vi "Set Protocol.vi"(8 "error in (no error)":errorcluster, 10 "protocol":refnum<class "Protocol Parent.lvclass">, 11 "instrument addon refnum in":T1 format="%.0x") -> (0 "error out":errorcluster, 3 "instrument addon refnum out":T1=18446744073709551615 format="%.0x")   [LabVIEW 2020, in "Instrument Addon Scripting API.lvlib"]
doc: "Sets the protocol object for the specified Instrument Addon Custom Device.\n \nThe input protocol must be a child of the protocol's parent class. It is formatted as one of the following classes: TCP.lvclass, UDP.lvclass, VISA.lvclass, RS-xxx.lvclass, AK TCP.lvclass, AK RS-xxx.lvclass, RS-xxx to GPIB ConvBox.lvclass"
uses:
  Instrument Addon Scripting API.lvlib
  <vilib>/NI VeriStand/Custom Device API/Custom Device Item Ref.ctl
  Libraries Directory/Protocols.lvlibp/Protocol Parent/Protocol Parent.lvclass
  Libraries Directory/Protocols.lvlibp/RS-xxx/RS-xxx.lvclass
  Shared Directory/RSXXX Port Settings.ctl
  Shared Directory/FG Control.ctl
  Libraries Directory/Protocols.lvlibp/AK RS-xxx/AK RS-xxx.lvclass
  Libraries Directory/Protocols.lvlibp/UDP/UDP.lvclass
  Shared Directory/UDP Settings.ctl
  Libraries Directory/Protocols.lvlibp/TCP/TCP.lvclass
  Shared Directory/TCPIP Settings.ctl
  Libraries Directory/Protocols.lvlibp/AK TCP/AK TCP.lvclass
  Libraries Directory/Protocols.lvlibp/VISA/VISA.lvclass
  Shared Directory/VISA Settings.ctl
  Libraries Directory/Protocols.lvlibp/RS-xxx to GPIB ConvBox/RS-xxx to GPIB ConvBox.lvclass
  Shared Directory/GPIB ConvBox Settings.ctl
  Libraries Directory/Protocols.lvlibp/RS-xxx/Data Access/Read PortSettings.vi
  Shared Directory/Constants.vi
  <vilib>/NI VeriStand/Custom Device API/NI VeriStand - Get Item Property.vi
  <vilib>/NI VeriStand/Custom Device API/Get Item Property (String).vi
  <vilib>/NI VeriStand/Custom Device API/Get Item Property (U32).vi
  <vilib>/NI VeriStand/Custom Device API/Get Item Property (Boolean).vi
  <vilib>/NI VeriStand/Custom Device API/NI VeriStand - Set Item Property.vi
  <vilib>/NI VeriStand/Custom Device API/Set Item Property (String).vi
  <vilib>/NI VeriStand/Custom Device API/Set Item Property (U32).vi
  <vilib>/NI VeriStand/Custom Device API/Set Item Property (Boolean).vi
  Dependencies.llb/Instrument_Addon_Scripting_Dependencies_SysDef.Property.Get.vi
  Dependencies.llb/Instrument_Addon_Scripting_Dependencies_SysDef.Property.Get.String.vi
  Dependencies.llb/Instrument_Addon_Scripting_Dependencies_SysDef.Property.Set.vi
  Dependencies.llb/Instrument_Addon_Scripting_Dependencies_SysDef.Property.Set.String.vi
  Libraries Directory/Protocols.lvlibp/UDP/Data Access/Read Local IP Address.vi
  Libraries Directory/Protocols.lvlibp/UDP/Data Access/Read Local Port.vi
  Libraries Directory/Protocols.lvlibp/UDP/Data Access/Read Target IP Address.vi
  Libraries Directory/Protocols.lvlibp/UDP/Data Access/Read Target Port.vi
  Libraries Directory/Protocols.lvlibp/TCP/Data Access/Read IP Address.vi
  Libraries Directory/Protocols.lvlibp/TCP/Data Access/Read Port.vi
  Libraries Directory/Protocols.lvlibp/VISA/Data Access/Read Append Write Termination Character.vi
  Libraries Directory/Protocols.lvlibp/VISA/Data Access/Read Enable Termination Character.vi
  Libraries Directory/Protocols.lvlibp/VISA/Data Access/Read Termination Character.vi
  Libraries Directory/Protocols.lvlibp/VISA/Data Access/Read Timeout.vi
  Libraries Directory/Protocols.lvlibp/VISA/Data Access/Read VISA Resource.vi
  Libraries Directory/Protocols.lvlibp/RS-xxx to GPIB ConvBox/Data Access/Read Assert Ren with IFC.vi
  Libraries Directory/Protocols.lvlibp/RS-xxx to GPIB ConvBox/Data Access/Read ConvBox Address.vi
  Libraries Directory/Protocols.lvlibp/RS-xxx to GPIB ConvBox/Data Access/Read GPIB Address.vi
  Libraries Directory/Protocols.lvlibp/RS-xxx to GPIB ConvBox/Data Access/Read IST bit sense.vi
  Libraries Directory/Protocols.lvlibp/RS-xxx to GPIB ConvBox/Data Access/Read Port.vi
  Libraries Directory/Protocols.lvlibp/RS-xxx to GPIB ConvBox/Data Access/Read System controller.vi
  Shared Directory/Instrument Addon Shared.lvlib
  <vilib>/NI VeriStand/Custom Device API/Custom Device API.lvlib
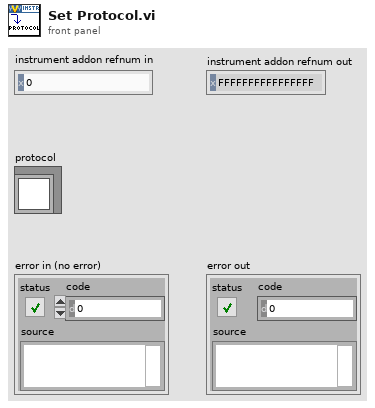
[diagram p1: front panel]
types:
  T1 = typedef "Custom Device API.lvlib/Custom Device Item Ref.ctl" = u64
  T2 = typedef "Instrument Addon Shared.lvlib/FG Control.ctl" = enum16{"Get", "Set"}
  T3 = typedef "Instrument Addon Shared.lvlib/RSXXX Port Settings.ctl" = cluster{"Port":string, "Baud Rate":u32, "Data Bits":u16, "Parity":enum16{"None", "Odd", "Even", "Mark", "Space"}, "Stop Bits":u16, "Flow Control":u16, "XON":enum16{"NUL", "SOH", "STX", "ETX", "EOT", "ENQ", "ACK", "BEL", "BS", "HT", "LF", "VT", "FF", "CR", "SO", "SI", "DLE", "DC1", "DC2", "DC3", "DC4", "NAK", "SYN", "ETB", "CAN", "EM", "SUB", "ESC", "FS", "GS", "RS", "US", "SP", "!", "\"", "#", "$", "%", "&", "'", "(", ")", "*", "+", ",", "- (-)", ".", "/", "0", "1", "2", "3", "4", "5", "6", "7", "8", "9", ":", ";", "<", "=", ">", "?", "@", "A", "B", "C", "D", "E", "F", "G", "H", "I", "J", "K", "L", "M", "N", "O", "P", "Q", "R", "S", "T", "U", "V", "W", "X", "Y", "Z", "[", "\\", "]", "^", "_", "`", "a", "b", "c", "d", "e", "f", "g", "h", "i", "j", "k", "l", "m", "n", "o", "p", "q", "r", "s", "t", "u", "v", "w", "x", "y", "z", "{", "|", "}", "~"}, "XOFF":enum16{"NUL", "SOH", "STX", "ETX", "EOT", "ENQ", "ACK", "BEL", "BS", "HT", "LF", "VT", "FF", "CR", "SO", "SI", "DLE", "DC1", "DC2", "DC3", "DC4", "NAK", "SYN", "ETB", "CAN", "EM", "SUB", "ESC", "FS", "GS", "RS", "US", "SP", "!", "\"", "#", "$", "%", "&", "'", "(", ")", "*", "+", ",", "- (-)", ".", "/", "0", "1", "2", "3", "4", "5", "6", "7", "8", "9", ":", ";", "<", "=", ">", "?", "@", "A", "B", "C", "D", "E", "F", "G", "H", "I", "J", "K", "L", "M", "N", "O", "P", "Q", "R", "S", "T", "U", "V", "W", "X", "Y", "Z", "[", "\\", "]", "^", "_", "`", "a", "b", "c", "d", "e", "f", "g", "h", "i", "j", "k", "l", "m", "n", "o", "p", "q", "r", "s", "t", "u", "v", "w", "x", "y", "z", "{", "|", "}", "~"}, "End Read on Termination Character":bool, "End Write on Termination Character":bool, "Termination Character":u8}
  T4 = typedef "Instrument Addon Shared.lvlib/UDP Settings.ctl" = cluster{"Local IP Address":string, "Local Port":u16, "Target IP Address":string, "Target Port":u16}
  T5 = typedef "Instrument Addon Shared.lvlib/TCPIP Settings.ctl" = cluster{"IP Address":string, "Port":u16}
  T6 = typedef "Instrument Addon Shared.lvlib/VISA Settings.ctl" = cluster{"VISA Resource":string, "Enable Termination Character":bool, "Termination Character":u8, "Timeout":u32, "Append Write Termination Character":bool}
  T7 = typedef "Instrument Addon Shared.lvlib/GPIB ConvBox Settings.ctl" = cluster{"Port":string, "ConvBox Address":string, "Assert Ren with IFC":bool, "System controller":bool, "IST bit sense":bool, "GPIB Address":string}
  T8 = typedef "Protocols.lvlibp/Protocol Parent.lvclass/Base Protocol Type.ctl" = enum16{"RS-XXX", "VISA", "TCPIP", "UDP", "GPIB ConvBox"}
  T9 = cluster{"Port":string, "Baud Rate":u32, "Data Bits":u16, "Parity":enum16{"None", "Odd", "Even", "Mark", "Space"}, "Stop Bits":u16, "Flow Control":u16, "XON":enum16{"NUL", "SOH", "STX", "ETX", "EOT", "ENQ", "ACK", "BEL", "BS", "HT", "LF", "VT", "FF", "CR", "SO", "SI", "DLE", "DC1", "DC2", "DC3", "DC4", "NAK", "SYN", "ETB", "CAN", "EM", "SUB", "ESC", "FS", "GS", "RS", "US", "SP", "!", "\"", "#", "$", "%", "&", "'", "(", ")", "*", "+", ",", "- (-)", ".", "/", "0", "1", "2", "3", "4", "5", "6", "7", "8", "9", ":", ";", "<", "=", ">", "?", "@", "A", "B", "C", "D", "E", "F", "G", "H", "I", "J", "K", "L", "M", "N", "O", "P", "Q", "R", "S", "T", "U", "V", "W", "X", "Y", "Z", "[", "\\", "]", "^", "_", "`", "a", "b", "c", "d", "e", "f", "g", "h", "i", "j", "k", "l", "m", "n", "o", "p", "q", "r", "s", "t", "u", "v", "w", "x", "y", "z", "{", "|", "}", "~"}, "XOFF":enum16{"NUL", "SOH", "STX", "ETX", "EOT", "ENQ", "ACK", "BEL", "BS", "HT", "LF", "VT", "FF", "CR", "SO", "SI", "DLE", "DC1", "DC2", "DC3", "DC4", "NAK", "SYN", "ETB", "CAN", "EM", "SUB", "ESC", "FS", "GS", "RS", "US", "SP", "!", "\"", "#", "$", "%", "&", "'", "(", ")", "*", "+", ",", "- (-)", ".", "/", "0", "1", "2", "3", "4", "5", "6", "7", "8", "9", ":", ";", "<", "=", ">", "?", "@", "A", "B", "C", "D", "E", "F", "G", "H", "I", "J", "K", "L", "M", "N", "O", "P", "Q", "R", "S", "T", "U", "V", "W", "X", "Y", "Z", "[", "\\", "]", "^", "_", "`", "a", "b", "c", "d", "e", "f", "g", "h", "i", "j", "k", "l", "m", "n", "o", "p", "q", "r", "s", "t", "u", "v", "w", "x", "y", "z", "{", "|", "}", "~"}, "End Read on Termination Character":bool, "End Write on Termination Character":bool, "Termination Character":u8}
  T10 = enum16{"NUL", "SOH", "STX", "ETX", "EOT", "ENQ", "ACK", "BEL", "BS", "HT", "LF", "VT", "FF", "CR", "SO", "SI", "DLE", "DC1", "DC2", "DC3", "DC4", "NAK", "SYN", "ETB", "CAN", "EM", "SUB", "ESC", "FS", "GS", "RS", "US", "SP", "!", "\"", "#", "$", "%", "&", "'", "(", ")", "*", "+", ",", "- (-)", ".", "/", "0", "1", "2", "3", "4", "5", "6", "7", "8", "9", ":", ";", "<", "=", ">", "?", "@", "A", "B", "C", "D", "E", "F", "G", "H", "I", "J", "K", "L", "M", "N", "O", "P", "Q", "R", "S", "T", "U", "V", "W", "X", "Y", "Z", "[", "\\", "]", "^", "_", "`", "a", "b", "c", "d", "e", "f", "g", "h", "i", "j", "k", "l", "m", "n", "o", "p", "q", "r", "s", "t", "u", "v", "w", "x", "y", "z", "{", "|", "}", "~"}
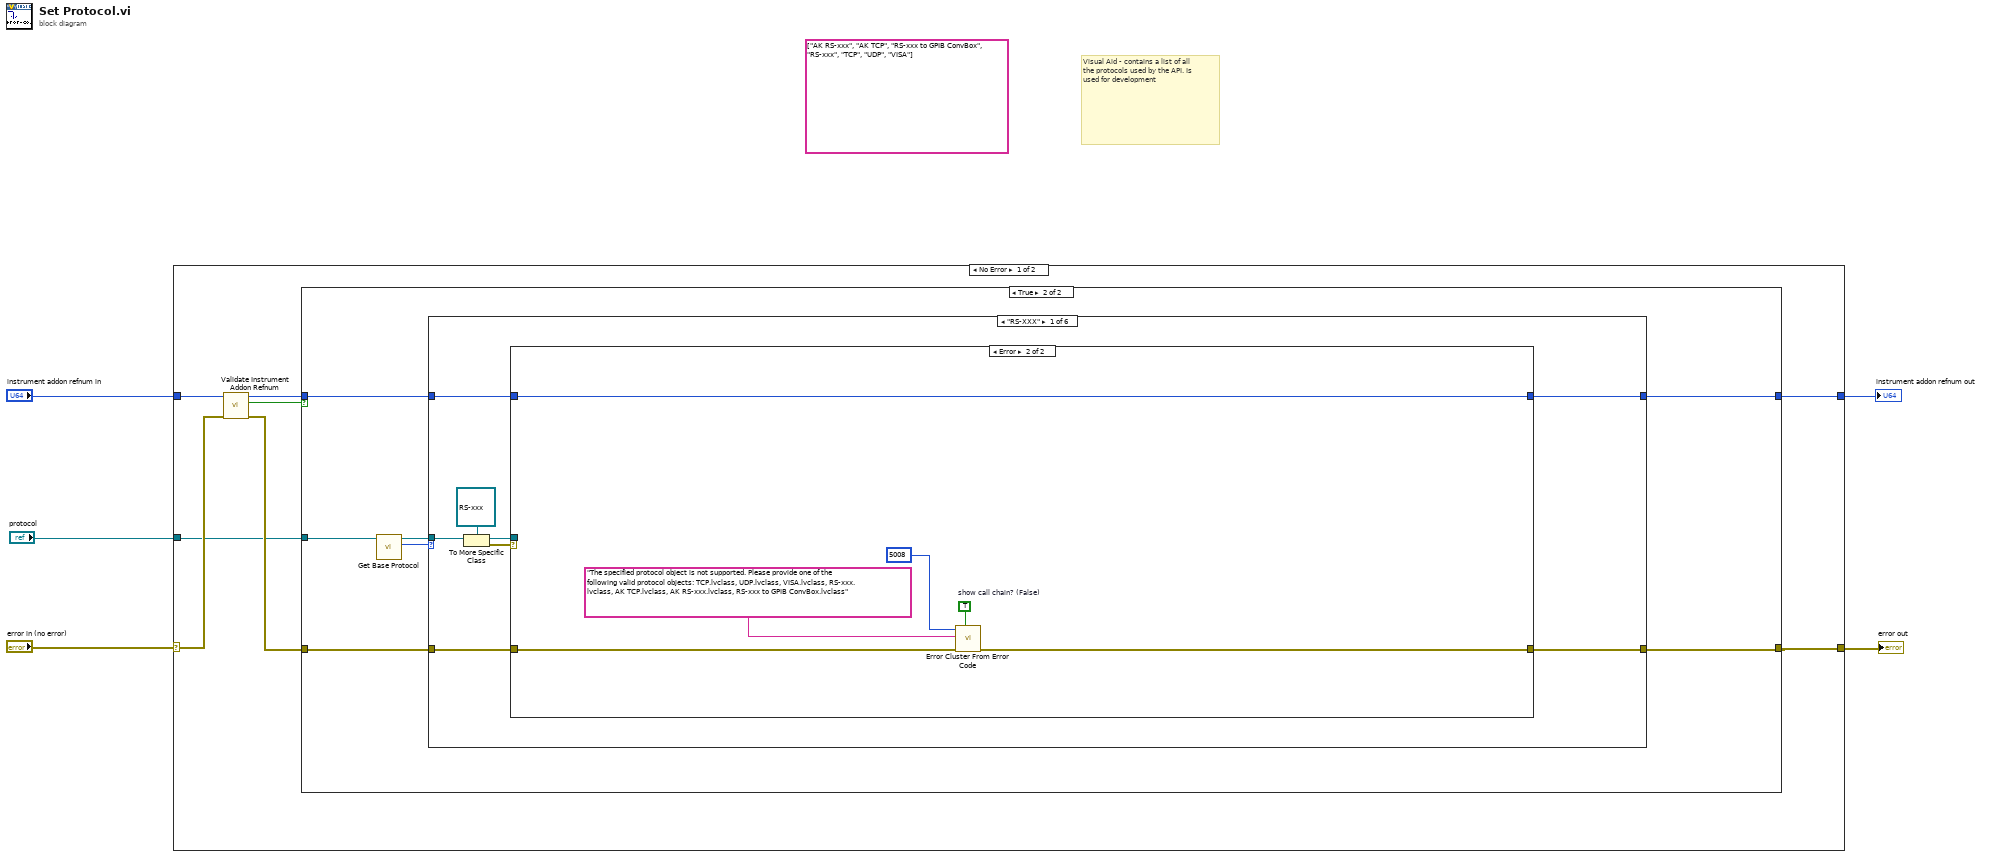
[diagram p0: block diagram]
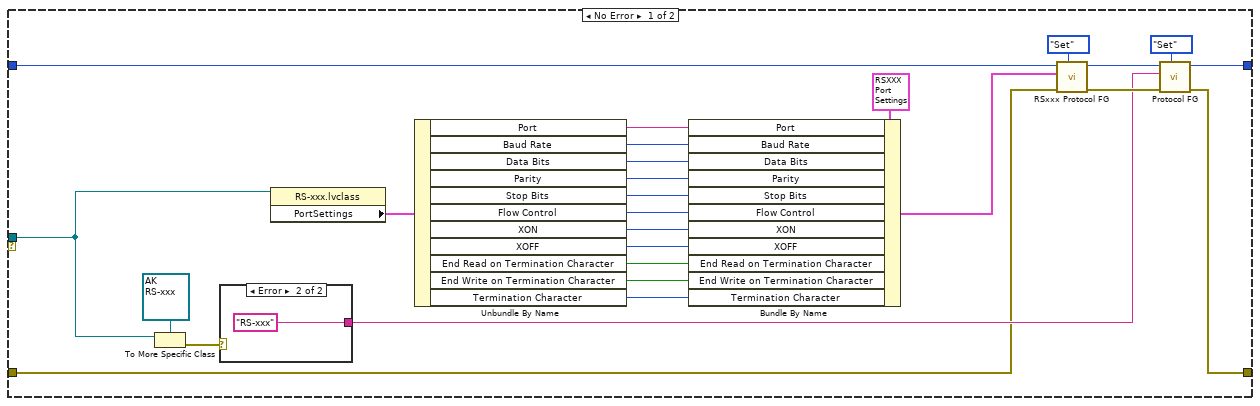
[diagram p3: hidden frame]
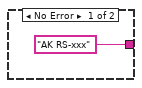
[diagram p4: hidden frame]
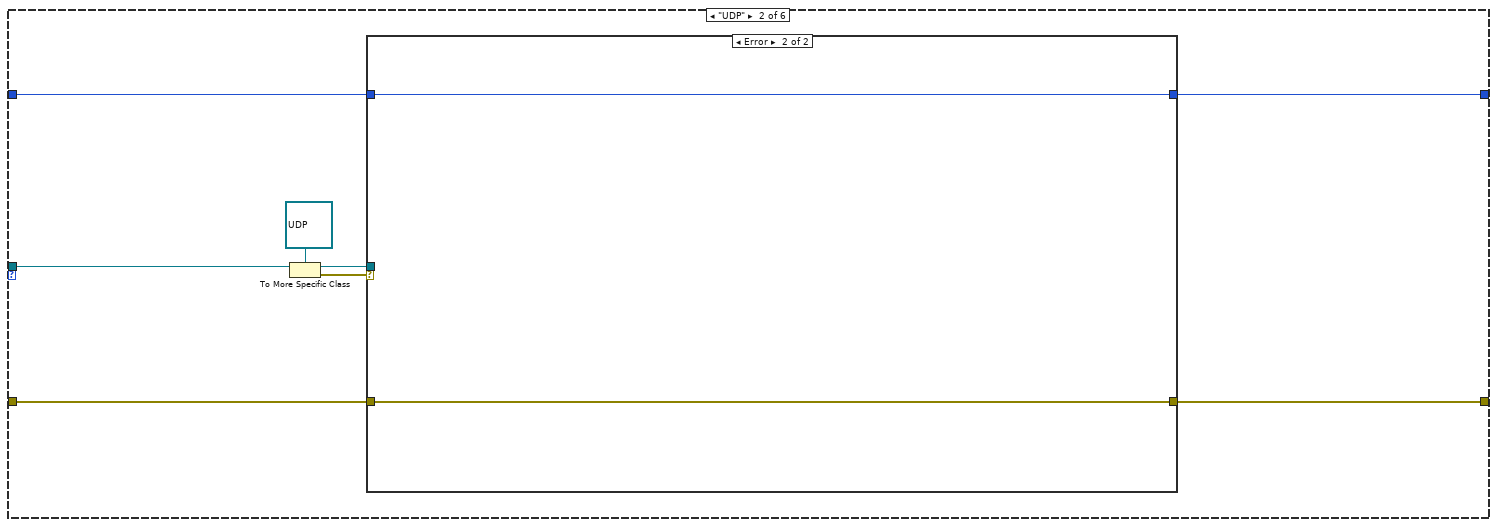
[diagram p5: hidden frame]
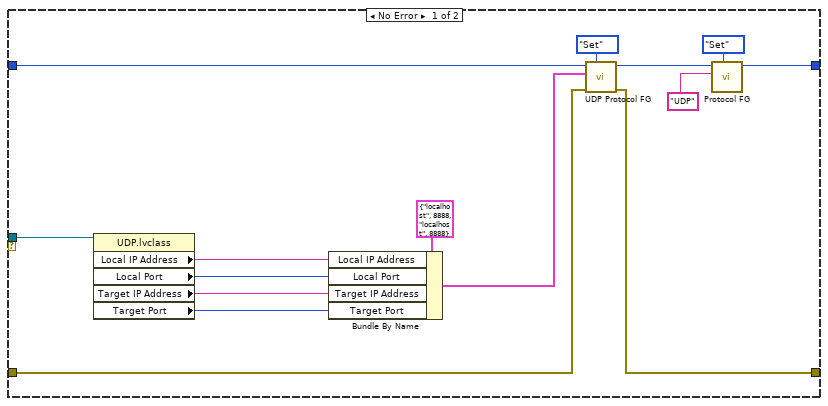
[diagram p6: hidden frame]
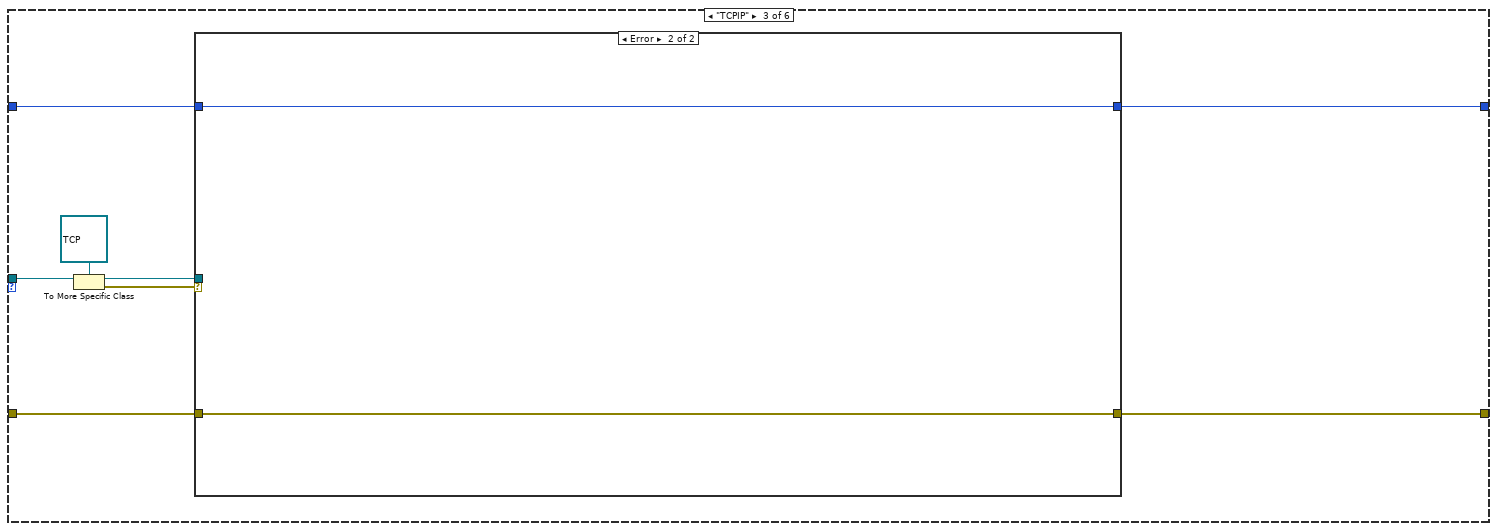
[diagram p7: hidden frame]
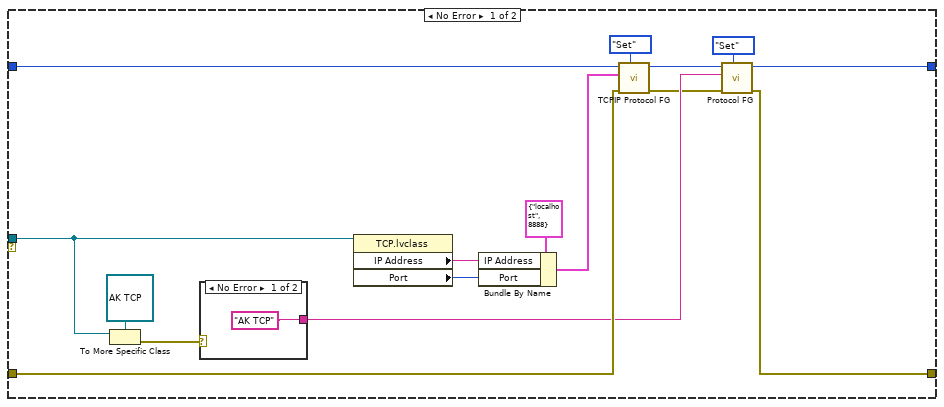
[diagram p8: hidden frame]
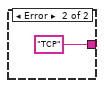
[diagram p9: hidden frame]
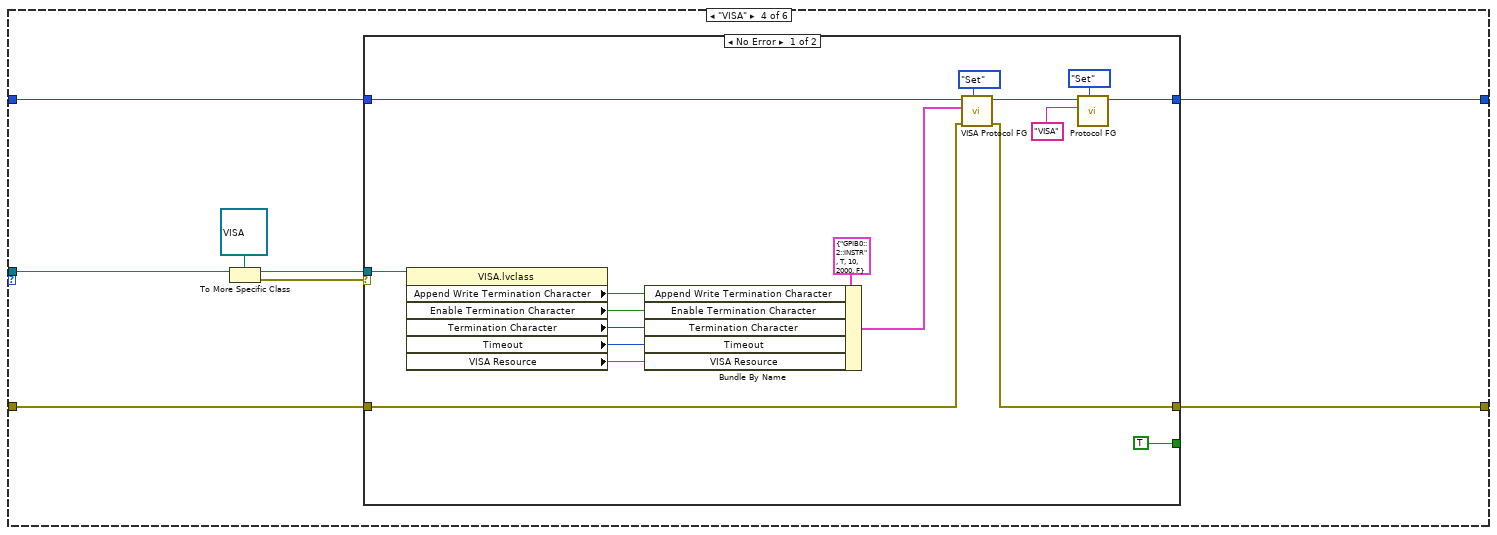
[diagram p10: hidden frame]
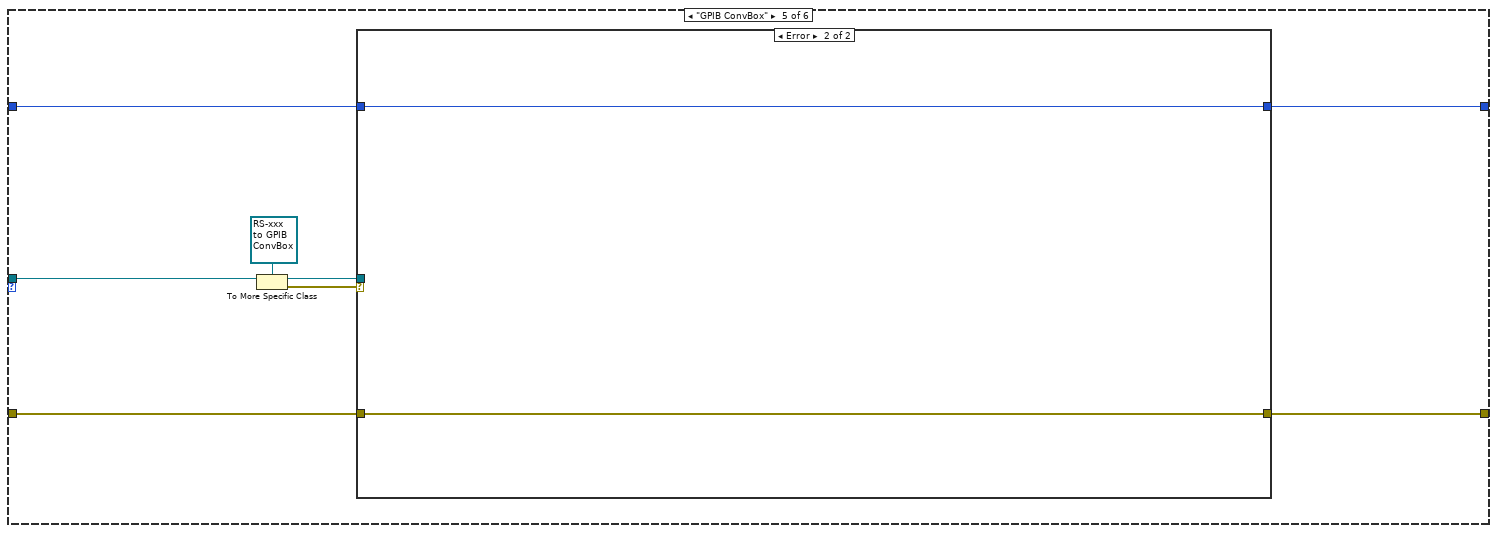
[diagram p12: hidden frame]
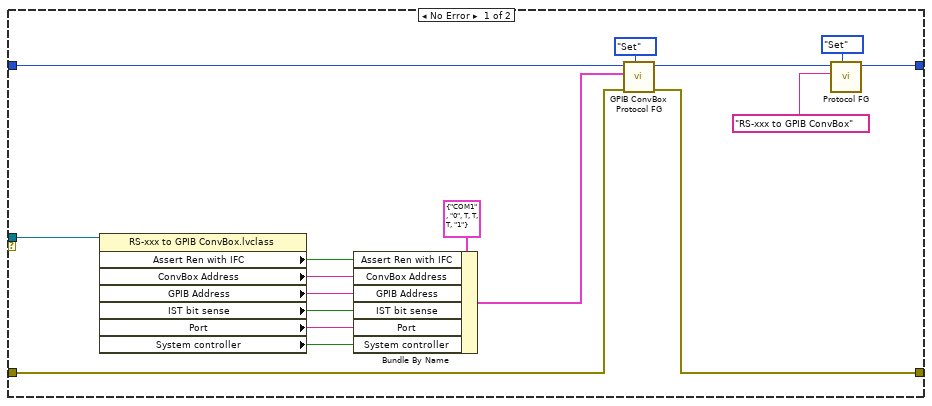
[diagram p13: hidden frame]
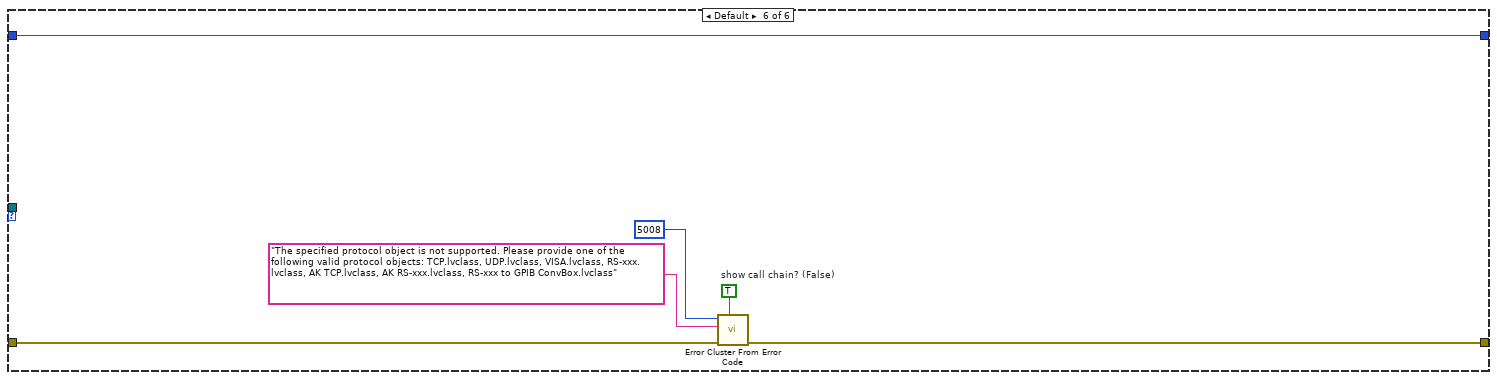
[diagram p14: hidden frame]
diagram:
  (unwired) string[] ["AK RS-xxx", "AK TCP", "RS-xxx to GPIB ConvBox", "RS-xxx", "TCP", "UDP", "VISA"] ("Array")
  # "Visual Aid - contains a list of all the protocols used by the API. Is used for development"
  n1 = case shown="No Error" "error in (no error)" {
    selector: "error in (no error)" -> [w12 w179]
    tunnel: "instrument addon refnum in" -> [w13 w178]
    tunnel: [w9 w179] -> w4
    tunnel: [w8 w178] -> w2
    tunnel: "protocol" -> [w6 _]
    frame No Error {
      n2 = call "Validate Instrument Addon Refnum.vi"("Error In"=w12, "Refnum In"=w13) -> ("Error Out"=w7:errorcluster, "Is Instrument Addon?"=w10:bool, "Refnum Out"=w11:T1)  [unwired: 7 in]
      n3 = case shown="True" w10 {
        tunnel: w11 -> [w15 w21]
        tunnel: [w14 w19] -> w9
        tunnel: [w15 w20] -> w8
        tunnel: w7 -> [w14 w22]
        tunnel: w6 -> [_ w18]
        frame False {
        }
        frame True {
          n4 = call-dynamic "Get Base Protocol.vi"("Protocol Parent in"=w18) -> ("Protocol out"=w16:T8, "Protocol Parent out"=w17:refnum<class "Protocol Parent.lvclass">)  [unwired: 8 in, 1 out]
          n5 = case shown="\"RS-XXX\"" w16 {
            tunnel: w17 -> [w29 w72 w97 w125 w152 _]
            tunnel: w22 -> [w24 w66 w91 w122 w148 w176]
            tunnel: w21 -> [w26 w70 w93 w121 w147 w177]
            tunnel: [w25 w69 w92 w119 w146 w177] -> w20
            tunnel: [w23 w65 w90 w118 w145 w173] -> w19
            frame "RS-XXX" {
              n6 = To More Specific Class(target class=refnum<class "RS-xxx.lvclass"> refnum ("Protocols.lvlibp:RS-xxx.lvclass"), reference=w29) -> (specific class reference=w27:refnum<class "RS-xxx.lvclass">, error out=w28:errorcluster)  [unwired: 1 in]
              n7 = case shown="Error" w28 {
                tunnel: w27 -> [w34 _]
                tunnel: w26 -> [w54 w64]
                tunnel: [w37 w64] -> w25
                tunnel: w24 -> [w31 w61]
                tunnel: [w36 w60] -> w23
                frame No Error {
                  n8 = To More Specific Class(target class=refnum<class "AK RS-xxx.lvclass"> refnum ("Protocols.lvlibp:AK RS-xxx.lvclass"), reference=w34) -> (error out=w33:errorcluster)  [unwired: 1 in, 1 out]
                  n9 = case shown="Error" w33 {
                    tunnel: ["AK RS-xxx" ("filename without extension") "RS-xxx" ("filename without extension")] -> w32
                    frame No Error {
                    }
                    frame Error {
                    }
                  }
                  n10 = property class="RS-xxx.lvclass"(reference=w34) -> ("PortSettings"=w55:T9)  [unwired: 1 in, 2 out]
                  n11 = Unbundle By Name(w55) -> ("Port"=w53:string, "Baud Rate"=w52:u32, "Data Bits"=w51:u16, "Parity"=w50:enum16{"None", "Odd", "Even", "Mark", "Space"}, "Stop Bits"=w49:u16, "Flow Control"=w48:u16, "XON"=w47:T10, "XOFF"=w46:T10, "End Read on Termination Character"=w45:bool, "End Write on Termination Character"=w44:bool, "Termination Character"=w43:u8)
                  n12 = Bundle By Name(cluster=T3 {"Port"="COM1", "Baud Rate"=9600, "Data Bits"=8, "Parity"=enum."None", "Stop Bits"=10, "Flow Control"=0, "XON"=enum."DC1", "XOFF"=enum."DC3", "End Read on Termination Character"=TRUE, "End Write on Termination Character"=TRUE, "Termination Character"=10} ("Serial Config"), "Port"=w53, "Baud Rate"=w52, "Data Bits"=w51, "Parity"=w50, "Stop Bits"=w49, "Flow Control"=w48, "XON"=w47, "XOFF"=w46, "End Read on Termination Character"=w45, "End Write on Termination Character"=w44, "Termination Character"=w43) -> (w41:T3)
                  n13 = call "RSxxx Protocol FG.vi"("Action"=FG_Control."Set", "error in (no error)"=w31, "Serial Config"=w41, "Device Item Ref in"=w54) -> ("error out"=w38:errorcluster, "Item Ref out"=w39:T1)  [unwired: 5 in, 1 out]
                  n14 = call "Protocol FG.vi"("Action"=FG_Control."Set", "error in (no error)"=w38, "Protocol"=w32, "Device Item Ref in"=w39) -> ("error out"=w36:errorcluster, "Item Ref out"=w37:T1)  [unwired: 5 in, 1 out]
                }
                frame Error {
                  w59 = TRUE  # show call chain? (False)
                  n15 = call <vilib>:"Error Cluster From Error Code.vi"("show call chain? (False)"=w59, "error in (no error)"=w61, "error message (\"\")"="The specified protocol object is not supported. Please provide one of the following valid protocol objects: TCP.lvclass, UDP.lvclass, VISA.lvclass, RS-xxx.lvclass, AK TCP.lvclass, AK RS-xxx.lvclass, RS-xxx to GPIB ConvBox.lvclass" ("error message (\"\")"), "error code (0)"=5008) -> ("error out"=w60:errorcluster)  [unwired: 5 in]
                }
              }
            }
            frame "UDP" {
              n16 = To More Specific Class(target class=refnum<class "UDP.lvclass"> refnum ("Protocols.lvlibp:UDP.lvclass"), reference=w72) -> (specific class reference=w67:refnum<class "UDP.lvclass">, error out=w68:errorcluster)  [unwired: 1 in]
              n17 = case shown="Error" w68 {
                tunnel: w70 -> [w87 w89]
                tunnel: [w74 w89] -> w69
                tunnel: w67 -> [w85 _]
                tunnel: w66 -> [w78 w88]
                tunnel: [w77 w88] -> w65
                frame No Error {
                  n18 = property class="UDP.lvclass"(reference=w85) -> ("Local IP Address"=w83:string, "Local Port"=w82:u16, "Target IP Address"=w81:string, "Target Port"=w80:u16)  [unwired: 1 in, 2 out]
                  n19 = Bundle By Name(cluster=T4 {"Local IP Address"="localhost", "Local Port"=8888, "Target IP Address"="localhost", "Target Port"=8888} ("UDP Config"), "Local IP Address"=w83, "Local Port"=w82, "Target IP Address"=w81, "Target Port"=w80) -> (w79:T4)
                  n20 = call "UDP Protocol FG.vi"("Action"=FG_Control."Set", "error in (no error)"=w78, "UDP Config"=w79, "Device Item Ref in"=w87) -> ("error out"=w77:errorcluster, "Item Ref out"=w75:T1)  [unwired: 5 in, 1 out]
                  n21 = call "Protocol FG.vi"("Action"=FG_Control."Set", "Protocol"="UDP" ("Local IP Address"), "Device Item Ref in"=w75) -> ("Item Ref out"=w74:T1)  [unwired: 6 in, 2 out]
                }
                frame Error {
                }
              }
            }
            frame "TCPIP" {
              n22 = To More Specific Class(target class=refnum<class "TCP.lvclass"> refnum ("Protocols.lvlibp:TCP.lvclass"), reference=w97) -> (specific class reference=w94:refnum<class "TCP.lvclass">, error out=w95:errorcluster)  [unwired: 1 in]
              n23 = case shown="Error" w95 {
                tunnel: w94 -> [w104 _]
                tunnel: w93 -> [w108 w116]
                tunnel: [w101 w116] -> w92
                tunnel: w91 -> [w107 w117]
                tunnel: [w98 w117] -> w90
                frame No Error {
                  n24 = To More Specific Class(target class=refnum<class "AK TCP.lvclass"> refnum ("Protocols.lvlibp:AK TCP.lvclass"), reference=w104) -> (error out=w106:errorcluster)  [unwired: 1 in, 1 out]
                  n25 = case shown="No Error" w106 {
                    tunnel: ["AK TCP" ("filename without extension") "TCP" ("filename without extension")] -> w100
                    frame No Error {
                    }
                    frame Error {
                    }
                  }
                  n26 = property class="TCP.lvclass"(reference=w104) -> ("IP Address"=w111:string, "Port"=w110:u16)  [unwired: 1 in, 2 out]
                  n27 = Bundle By Name(cluster=T5 {"IP Address"="localhost", "Port"=8888} ("TCP/IP Config"), "IP Address"=w111, "Port"=w110) -> (w109:T5)
                  n28 = call "TCPIP Protocol FG.vi"("Action"=FG_Control."Set", "error in (no error)"=w107, "TCP/IP Config"=w109, "Device Item Ref in"=w108) -> ("error out"=w99:errorcluster, "Item Ref out"=w102:T1)  [unwired: 5 in, 1 out]
                  n29 = call "Protocol FG.vi"("Action"=FG_Control."Set", "error in (no error)"=w99, "Protocol"=w100, "Device Item Ref in"=w102) -> ("error out"=w98:errorcluster, "Item Ref out"=w101:T1)  [unwired: 5 in, 1 out]
                }
                frame Error {
                }
              }
            }
            frame "VISA" {
              n30 = To More Specific Class(target class=refnum<class "VISA.lvclass"> refnum ("Protocols.lvlibp:VISA.lvclass"), reference=w125) -> (specific class reference=w120:refnum<class "VISA.lvclass">, error out=w123:errorcluster)  [unwired: 1 in]
              n31 = case shown="No Error" w123 {
                tunnel: w122 -> [w131 w143]
                tunnel: w121 -> [w141 w144]
                tunnel: w120 -> [w142 _]
                tunnel: [w127 w144] -> w119
                tunnel: [TRUE _] -> _
                tunnel: [w130 w143] -> w118
                frame No Error {
                  n32 = property class="VISA.lvclass"(reference=w142) -> ("Append Write Termination Character"=w138:bool, "Enable Termination Character"=w137:bool, "Termination Character"=w136:u8, "Timeout"=w135:u32, "VISA Resource"=w134:string)  [unwired: 1 in, 2 out]
                  n33 = Bundle By Name(cluster=T6 {"VISA Resource"="GPIB0::2::INSTR", "Enable Termination Character"=TRUE, "Termination Character"=10, "Timeout"=2000, "Append Write Termination Character"=FALSE} ("VISA Config"), "Append Write Termination Character"=w138, "Enable Termination Character"=w137, "Termination Character"=w136, "Timeout"=w135, "VISA Resource"=w134) -> (w133:T6)
                  n34 = call "VISA Protocol FG.vi"("Action"=FG_Control."Set", "error in (no error)"=w131, "VISA Config"=w133, "Device Item Ref in"=w141) -> ("error out"=w130:errorcluster, "Item Ref out"=w128:T1)  [unwired: 5 in, 1 out]
                  n35 = call "Protocol FG.vi"("Action"=FG_Control."Set", "Protocol"="VISA", "Device Item Ref in"=w128) -> ("Item Ref out"=w127:T1)  [unwired: 6 in, 2 out]
                }
                frame Error {
                }
              }
            }
            frame "GPIB ConvBox" {
              n36 = To More Specific Class(target class=refnum<class "RS-xxx to GPIB ConvBox.lvclass"> refnum ("Protocols.lvlibp:RS-xxx to GPIB ConvBox.lvclass"), reference=w152) -> (specific class reference=w149:refnum<class "RS-xxx to GPIB ConvBox.lvclass">, error out=w150:errorcluster)  [unwired: 1 in]
              n37 = case shown="Error" w150 {
                tunnel: w149 -> [w169 _]
                tunnel: w148 -> [w167 w171]
                tunnel: w147 -> [w158 w170]
                tunnel: [w153 w170] -> w146
                tunnel: [w157 w171] -> w145
                frame No Error {
                  n38 = property class="RS-xxx to GPIB ConvBox.lvclass"(reference=w169) -> ("Assert Ren with IFC"=w165:bool, "ConvBox Address"=w164:string, "GPIB Address"=w163:string, "IST bit sense"=w162:bool, "Port"=w161:string, "System controller"=w160:bool)  [unwired: 1 in, 2 out]
                  n39 = Bundle By Name(cluster=T7 {"Port"="COM1", "ConvBox Address"="0", "Assert Ren with IFC"=TRUE, "System controller"=TRUE, "IST bit sense"=TRUE, "GPIB Address"="1"} ("GPIB ConvBox Config"), "Assert Ren with IFC"=w165, "ConvBox Address"=w164, "GPIB Address"=w163, "IST bit sense"=w162, "Port"=w161, "System controller"=w160) -> (w159:T7)
                  n40 = call "GPIB ConvBox Protocol FG.vi"("Action"=FG_Control."Set", "error in (no error)"=w167, "GPIB ConvBox Config"=w159, "Device Item Ref in"=w158) -> ("error out"=w157:errorcluster, "Item Ref out"=w154:T1)  [unwired: 5 in, 1 out]
                  n41 = call "Protocol FG.vi"("Action"=FG_Control."Set", "Protocol"="RS-xxx to GPIB ConvBox", "Device Item Ref in"=w154) -> ("Item Ref out"=w153:T1)  [unwired: 6 in, 2 out]
                }
                frame Error {
                }
              }
            }
            frame Default {
              w172 = TRUE  # show call chain? (False)
              n42 = call <vilib>:"Error Cluster From Error Code.vi"("show call chain? (False)"=w172, "error in (no error)"=w176, "error message (\"\")"="The specified protocol object is not supported. Please provide one of the following valid protocol objects: TCP.lvclass, UDP.lvclass, VISA.lvclass, RS-xxx.lvclass, AK TCP.lvclass, AK RS-xxx.lvclass, RS-xxx to GPIB ConvBox.lvclass" ("error message (\"\")"), "error code (0)"=5008) -> ("error out"=w173:errorcluster)  [unwired: 5 in]
            }
          }
        }
      }
    }
    frame Error {
    }
  }
  "error out" <- w4
  "instrument addon refnum out" <- w2
